vi "Set Measurement Start Time.vi"(8 "error in (no error)":errorcluster, 10 "Time Stamp (now)":timestamp, 11 "BLF File In":refnum<class "Read Write BLF.lvclass">) -> (0 "error out":errorcluster, 3 "BLF File Out":refnum<class "Read Write BLF.lvclass">)   [LabVIEW 2015, in "Read Write BLF.lvclass"]
doc: "This VI will set the Start Time of the BLF file. By default this time is the current time and date. If this function is not ran when the first object is written, the start time will be set to the time of the first CAN Frame written.\n\n-------------\nBrian Hoover (Hooovahh)"
uses:
  Read Write BLF.lvclass
  Read Write BLF.lvclass/Read Write BLF.ctl
  Controls/Cluster - SystemTime.ctl
  <vilib>/Utility/error.llb/Error Cluster From Error Code.vi
  <vilib>/Utility/file.llb/Application Directory.vi
  <vilib>/ErrorRing/Error Ring.xnode
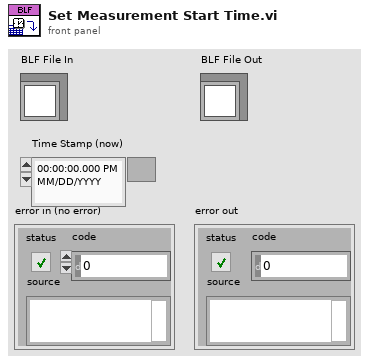
[diagram p1: front panel]
types:
  T1 = typedef "Read Write BLF.lvclass/Cluster - SystemTime.ctl" = cluster{"Year":u16, "Month":u16, "DayOfWeek":u16, "Day":u16, "Hour":u16, "Minute":u16, "Second":u16, "Milliseconds":u16}
  T2 = typedef "LVDateTimeRec.ctl" = cluster{"fractional second":dbl, "second":i32, "minute":i32, "hour":i32, "day of month":i32, "month":i32, "year":i32, "day of week":i32, "day of year":i32, "DST":i32}
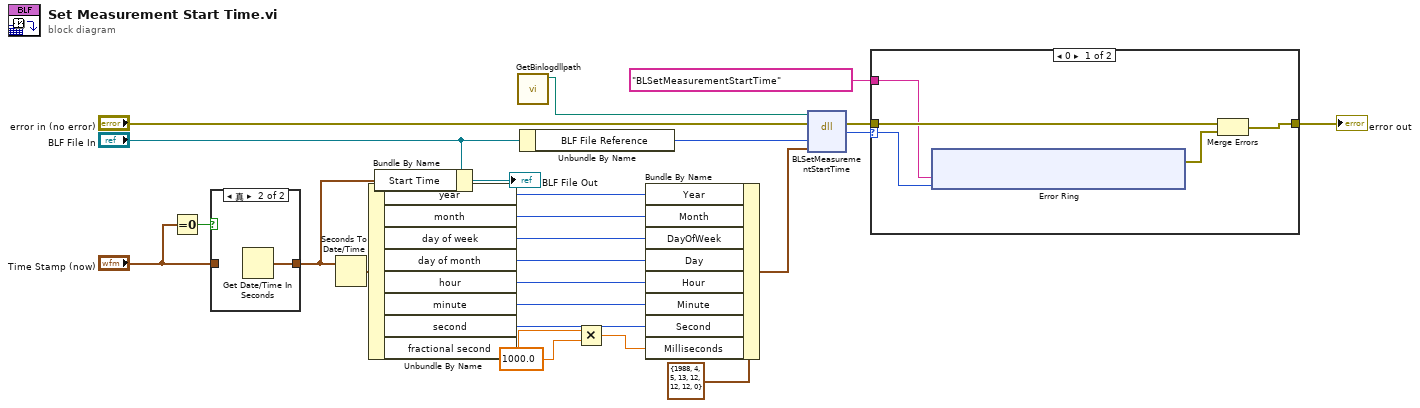
[diagram p0: block diagram]
diagram:
  n1 = Equal To 0?(x="Time Stamp (now)") -> (x = 0?=w4:bool)
  n2 = case shown="真" w4 {
    tunnel: "Time Stamp (now)" -> [w26 _]
    tunnel: [w26 w27] -> w2
    frame False {
    }
    frame True {
      n3 = Get Date/Time In Seconds() -> (seconds since 1Jan1904=w27:timestamp)
    }
  }
  n4 = Seconds To Date/Time(time stamp (now)=w2) -> (date time rec=w22:T2)  [unwired: 1 in]
  n5 = Unbundle By Name(w22) -> ("year"=w21:i32, "month"=w20:i32, "day of week"=w19:i32, "day of month"=w18:i32, "hour"=w17:i32, "minute"=w16:i32, "second"=w15:i32, "fractional second"=w14:dbl)
  n6 = Bundle By Name(cluster="BLF File In", "Start Time"=w2) -> (→"BLF File Out":refnum<class "Read Write BLF.lvclass">)
  n7 = call "GetBinlogdllpath.vi"() -> ("dup path"=w1:path)  [unwired: 11 in]
  n8 = Unbundle By Name("BLF File In") -> ("BLF File Reference"=w6:u32)
  n9 = Multiply(x=w14, y=1000.0) -> (x*y=w12:dbl)
  n10 = Bundle By Name(cluster=T1 {"Year"=1988, "Month"=4, "DayOfWeek"=5, "Day"=13, "Hour"=12, "Minute"=12, "Second"=12, "Milliseconds"=0} ("SYSTEMTIME"), "Year"=w21, "Month"=w20, "DayOfWeek"=w19, "Day"=w18, "Hour"=w17, "Minute"=w16, "Second"=w15, "Milliseconds"=w12) -> (w23:T1)
  n11 = dll-call lib="PTH2Vabs E自开发软件X-CAN项目 X-CAN离线分析平台 V2.2.8.0BLFbinlog.*" fn="BLSetMeasurementStartTime"(path in=w1, error in="error in (no error)", "hFile"=w6, "lpStartTime"=w23) -> (error out=w9:errorcluster, "return type"=w10:i32)  [unwired: 3 in, 1 out]
  n12 = case shown="0" w10 {
    selector: w10 -> [w30 _]
    tunnel: w9 -> [w32 w41]
    tunnel: [w31 w41] -> w8
    tunnel: "BLSetMeasurementStartTime" -> [w29 _]
    frame 0 {
      n13 = xnode "Error Ring"("参数 0"=w29, "参数 1"=w30) -> ("错误输出"=w28:errorcluster)
      n14 = Merge Errors(w32, w28) -> (w31:errorcluster)
    }
    frame Default {
    }
  }
  "error out" <- w8
